vi "Create_erase_jlink_file.vi"(1 "Password":string, 7 "path":path, 11 "error in":errorcluster) -> (15 "error out":errorcluster)   [LabVIEW 2023]
panel:
  # "s"
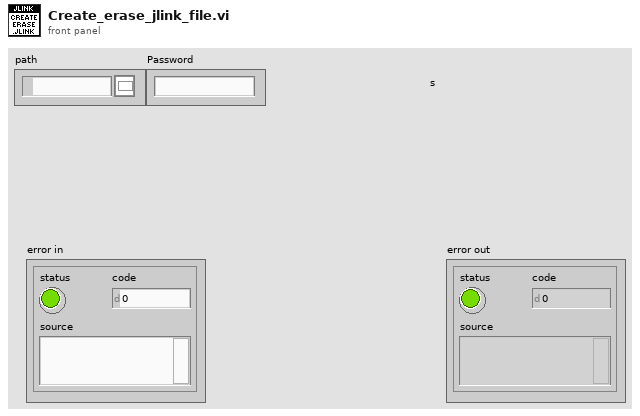
[diagram p1: front panel]
types:
  T1 = enum16{"open", "replace", "create", "open or create", "replace or create", "replace or create with confirmation"}
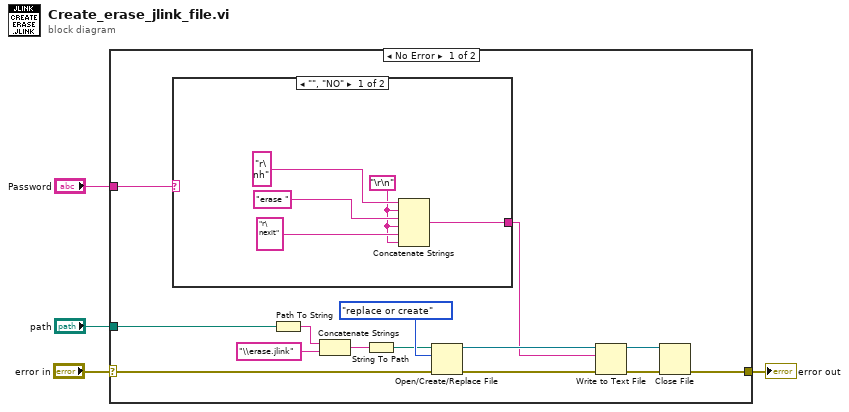
[diagram p0: block diagram]
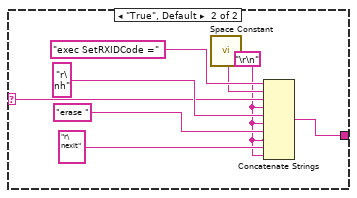
[diagram p2: hidden frame]
diagram:
  n1 = case shown="No Error" "error in" {
    selector: "error in" -> [w9 w32]
    tunnel: [w8 w32] -> w3
    tunnel: "Password" -> [w7 _]
    tunnel: "path" -> [w5 _]
    frame No Error {
      n2 = case shown="\"\", \"NO\"" w7 {
        selector: w7 -> [_ w26]
        tunnel: [w21 w29] -> w6
        frame "", "NO" {
          w19 = "\r\n"
          n3 = Concatenate Strings("r\nh" ("string"), w19, "erase " ("string"), w19, "r\nexit" ("string"), w19) -> (w21:string)
        }
        frame "True", Default {
          w24 = "\r\n"
          n4 = call <vilib>:"Space Constant.vi"() -> ("String"=w27:string)
          n5 = Concatenate Strings("exec SetRXIDCode =", w27, w26, w24, "r\nh" ("string"), w24, "erase " ("string"), w24, "r\nexit" ("string"), w24) -> (w29:string)
        }
      }
      n6 = Path To String(path=w5) -> (string=w11:string)
      n7 = Concatenate Strings(w11, "\\erase.jlink" ("string")) -> (w12:string)
      n8 = String To Path(string=w12) -> (path=w10:path)
      n9 = Open/Create/Replace File(file path (use dialog)=w10, error in=w9, operation (0:open)=T1."replace or create") -> (refnum out=w17:refnum<file>, error out=w16:errorcluster)  [unwired: 3 in, 1 out]
      n10 = Write to Text File(file (use dialog)=w17, text=w6, error in=w16) -> (refnum out=w15:refnum<file>, error out=w14:errorcluster)  [unwired: 1 in, 1 out]
      n11 = Close File(refnum=w15, error in=w14) -> (error out=w8:errorcluster)  [unwired: 1 out]
    }
    frame Error {
    }
  }
  "error out" <- w3
